vi "Get Refnum.vi"(8 "error in (no error)":errorcluster caption="entrée d'erreur (pas d'erreur)", 11 "Cryptographic Hash_SHA256 en entrée":refnum<class "Cryptographic Hash_SHA256.lvclass">) -> (0 "error out":errorcluster caption="sortie d'erreur", 2 "Refnum":refnum<k24>, 3 "Cryptographic Hash_SHA256 en sortie":refnum<class "Cryptographic Hash_SHA256.lvclass">)   [LabVIEW 2020, in "Library Cryptographic Hash.lvlib" / "Cryptographic Hash_SHA256.lvclass"]
uses:
  Cryptographic Hash_SHA256.lvclass
  Cryptographic Hash_SHA256.lvclass/Cryptographic Hash_SHA256.ctl
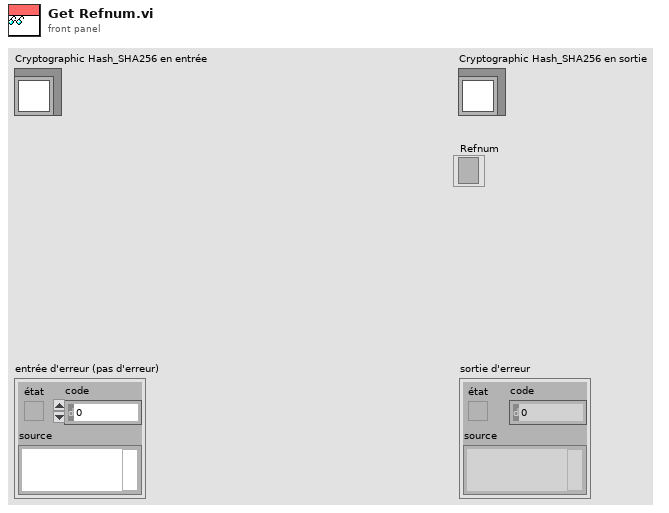
[diagram p1: front panel]
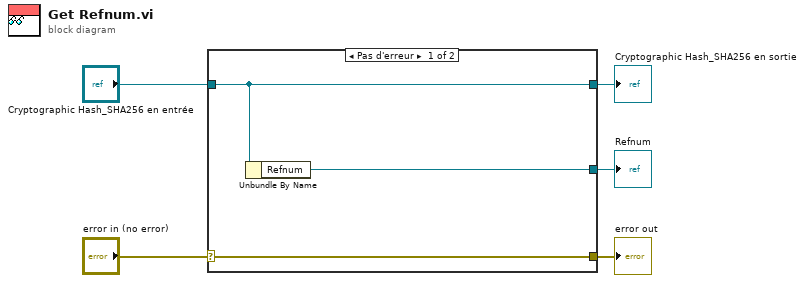
[diagram p0: block diagram]
diagram:
  n1 = case shown="Pas d'erreur" "error in (no error)" {
    selector: "error in (no error)" -> [w8 w9]
    tunnel: [w8 w9] -> w4
    tunnel: [w7 w10] -> w2
    tunnel: "Cryptographic Hash_SHA256 en entrée" -> [w7 w10]
    tunnel: [w6 _] -> w1
    frame No Error {
      n2 = Unbundle By Name(w7) -> ("Refnum"=w6:refnum<k24>)
    }
    frame Error {
    }
  }
  "error out" <- w4
  "Cryptographic Hash_SHA256 en sortie" <- w2
  "Refnum" <- w1
